vi "波形前面板显示.vi"(5 "X标尺.名称标签.文本":string="滴定数", 7 "标题.文本":string="滴定数-ORP值", 9 "ORP滴定曲线":u16[](graph), 10 "滴定数-ORP值":u16[](array[numeric]) caption="时间-温度", 11 "波形时间":timestamp) -> ()   [LabVIEW 2016, in "斯坦道CODMn.lvlib"]
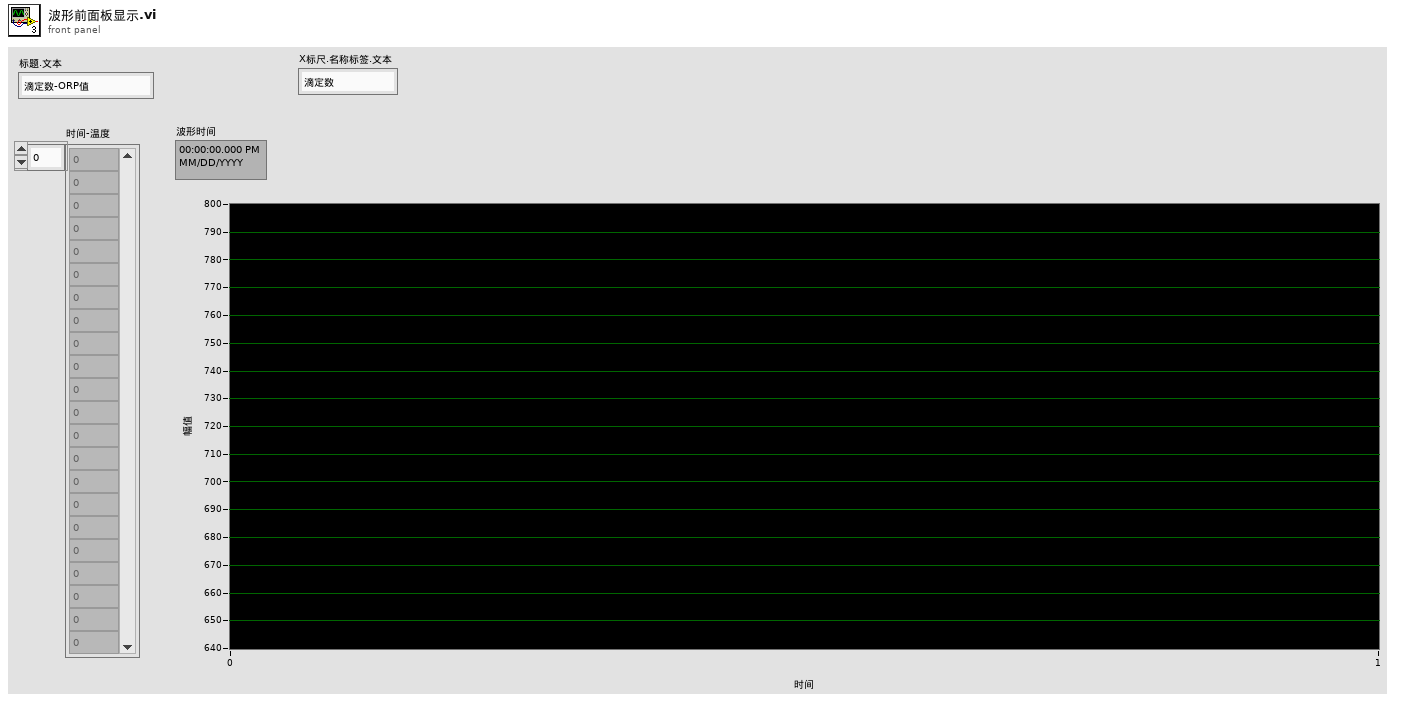
[diagram p1: front panel]
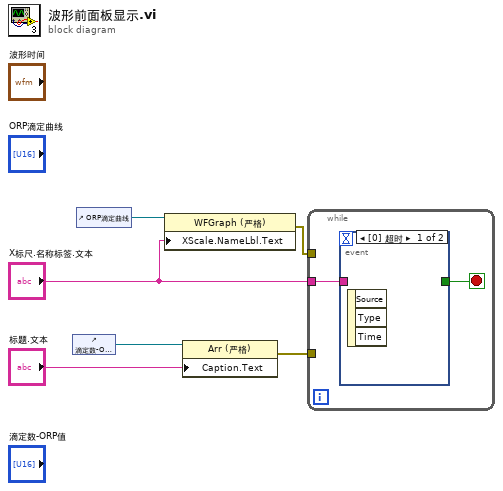
[diagram p0: block diagram]
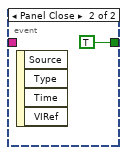
[diagram p2: hidden frame]
diagram:
  n1 = control-ref of="滴定数-ORP值"() -> (w6:refnum<vi>)
  n2 = control-ref of="ORP滴定曲线"() -> (w3:refnum<vi>)
  n3 = property class="WFGraph (严格)"(reference=w3, "XScale.NameLbl.Text"="X标尺.名称标签.文本") -> (error out=w2:errorcluster)  [unwired: 1 in, 1 out]
  n4 = property class="Arr (严格)"(reference=w6, "Caption.Text"="标题.文本") -> (error out=w4:errorcluster)  [unwired: 1 in, 1 out]
  n5 = while {
    tunnel: w4 -> [_]
    tunnel: w2 -> [_]
    tunnel: "X标尺.名称标签.文本" -> [w7]
    stop <- w8 stop-if-true
    n6 = event shown="[0] 超时" {
      selector: _ -> [_ _]
      dyn-events: _ -> [_ _]
      timeout: _ -> [_ _]
      tunnel: [_ TRUE] -> w8
      tunnel: w7 -> [_ _]
      event Timeout {
        n7 = event-data() -> ()  [unwired: 1 in, 3 out]
      }
      event Panel Close {
        n8 = event-data() -> ()  [unwired: 1 in, 4 out]
      }
    }
  }
